vi "Beat Sound.vi"() -> ()   [LabVIEW 2020]
doc: "This VI illustrates how to generate and play sine, square, sawtooth and triangle waveforms. You can change the frequency and type of the waveform generated as it plays continuously."
uses:
  <vilib>/sound2/lvsound2.llb/Sampling Mode.ctl
  <vilib>/sound2/lvsound2.llb/Sound Data Format.ctl
  <vilib>/sound2/lvsound2.llb/Sound Output Set Volume (Single).vi
  <vilib>/sound2/lvsound2.llb/Sound Output Write (DBL Single).vi
panel:
  in  "Frequency\nDifference [Hz]":dbl(slide)=0.6000000000000003 min=-10.0 max=10.0 step=0.1 scale=0.0..5.0
  in  "Volume":dbl(slide)=21.338912133891213 scale=0.0..100.0
  out "Generated Sound":waveform(dbl)[](graph)=[{"t0"=timestamp(29.931972789115648 s since 1904-01-01), "dt"=2.2675736961451248e-05, "Y"=array[10000 elements], "attributes"=variant("NI_ChannelName"=variant(string "Signal 1"), "NI_ExpIsRelativeTime"=variant(bool TRUE), "NI_ExpStartTimeStamp"=variant(timestamp timestamp(3695136105.7761874 s since 1904-01-01)), "NI_ExpTimeStamp"=variant(timestamp timestamp(3695136135.7081604 s since 1904-01-01)), "NI_ExpXDimension"=variant(string "t"))}, {"t0"=timestamp(29.931972789115648 s since 1904-01-01), "dt"=2.2675736961451248e-05, "Y"=array[10000 elements], "attributes"=variant("NI_ChannelName"=variant(string "Signal 2"), "NI_ExpIsRelativeTime"=variant(bool TRUE), "NI_ExpStartTimeStamp"=variant(timestamp timestamp(3695136105.777132 s since 1904-01-01)), "NI_ExpTimeStamp"=variant(timestamp timestamp(3695136135.709105 s since 1904-01-01)), "NI_ExpXDimension"=variant(string "t"))}, {"t0"=timestamp(29.931972789115648 s since 1904-01-01), "dt"=2.2675736961451248e-05, "Y"=array[10000 elements], "attributes"=variant("NI_ChannelName"=variant(string "Signal 1"), "NI_ExpIsRelativeTime"=variant(bool TRUE), "NI_ExpStartTimeStamp"=variant(timestamp timestamp(3695136105.7761874 s since 1904-01-01)), "NI_ExpTimeStamp"=variant(timestamp timestamp(3695136135.7081604 s since 1904-01-01)), "NI_ExpXDimension"=variant(string "t"))}]
  in  "Frequency [Hz]":dbl=440.0
  in  "Stop":bool
  # "Beat Tone Demo"
  # "McClellan et al., DSP First 3-2 Beat Notes"
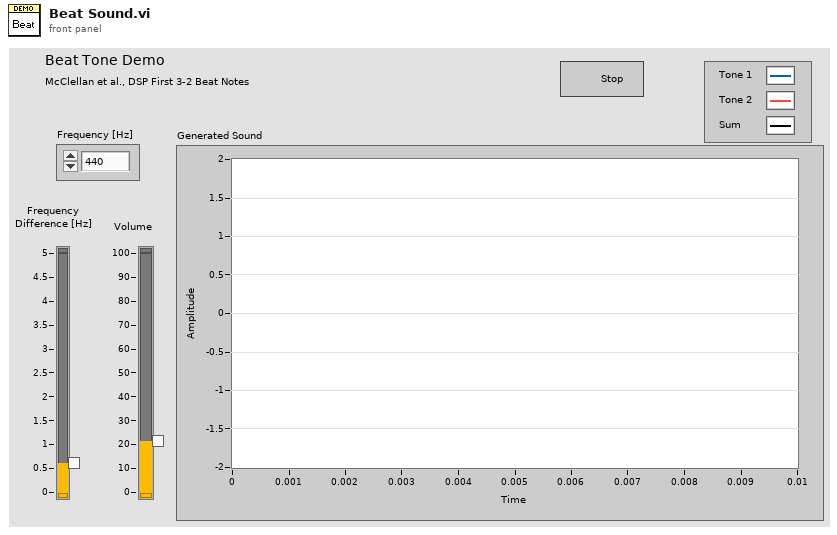
[diagram p1: front panel]
types:
  T1 = typedef "Sound Data Format.ctl" = cluster{"sample rate (S/s)":dbl, "number of channels":i32, "bits per sample":i32}
  T2 = typedef "Sampling Mode.ctl" = i32
  T3 = typedef "Sound Output Task ID.ctl" = u32
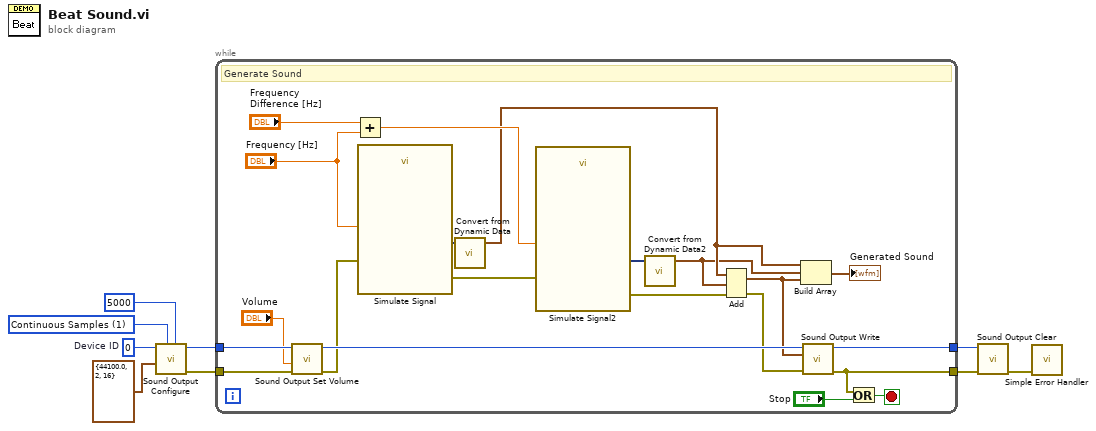
[diagram p0: block diagram]
diagram:
  w5 = u32 0  # Device ID
  w4 = T2 1 items=["Finite Samples", "Continuous Samples"] ("sample mode")
  n1 = call <vilib>:"Sound Output Configure.vi"("number of samples/ch"=5000 ("Number of Samples/ch"), "sample mode"=w4, "sound format"=T1 {"sample rate (S/s)"=44100.0, "number of channels"=2, "bits per sample"=16} ("Sound Format"), "device ID"=w5) -> ("error out"=w9:errorcluster, "task ID"=w8:T3)  [unwired: 6 in]
  n2 = while {
    tunnel: w8 -> [w25]
    tunnel: [w30] -> w6
    tunnel: w9 -> [w27]
    tunnel: [w23] -> w7
    stop <- w28 stop-if-true
    # "Generate Sound"
    n3 = call-poly <vilib>:"Sound Output Set Volume.vi"("error in (no error)"=w27, "volume"="Volume", "task ID"=w25) -> ("error out"=w22:errorcluster, "task ID out"=w26:T3)  [unwired: 7 in]
    n4 = Add(x="Frequency\nDifference [Hz]", y="Frequency [Hz]") -> (x+y=w17:dbl)
    n5 = call "Simulate Signal"("Frequency"="Frequency [Hz]", "error in (no error)"=w22) -> ("Signal 1"=w21:dynamicdata, "error out"=w20:errorcluster)  [unwired: 12 in]
    n6 = call "Convert from Dynamic Data"("Dynamic Data Type"=w21) -> ("Waveform"=w11:waveform(dbl))  [unwired: 3 in]
    n7 = call "Simulate Signal2"("Frequency"=w17, "error in (no error)"=w20) -> ("Signal 2"=w16:dynamicdata, "error out"=w15:errorcluster)  [unwired: 12 in]
    n8 = call "Convert from Dynamic Data2"("Dynamic Data Type"=w16) -> ("Waveform"=w10:waveform(dbl))  [unwired: 3 in]
    n9 = Add(1:w10, 2:w11, 4:w15) -> (0:w13:waveform(dbl), 3:w14:errorcluster)
    n10 = Build Array(w11, w10, w13) -> (→"Generated Sound":waveform(dbl)[])
    n11 = call-poly <vilib>:"Sound Output Write.vi"("error in (no error)"=w14, "data"=w13, "task ID"=w26) -> ("error out"=w23:errorcluster, "task ID out"=w30:T3)  [unwired: 7 in]
    n12 = Or(x=w23, y="Stop") -> (x .or. y?=w28:bool)
  }
  n13 = call <vilib>:"Sound Output Clear.vi"("error in (no error)"=w7, "task ID"=w6) -> ("error out"=w2:errorcluster)  [unwired: 9 in]
  n14 = call <vilib>:"Simple Error Handler.vi"("error in (no error)"=w2) -> ()  [unwired: 4 in, 5 out]
